vi "set current selections.vi"   [LabVIEW 2017, in "vs-tree-utility.lvlib" / "alias-tree.lvclass"]
uses:
  alias-tree.lvclass
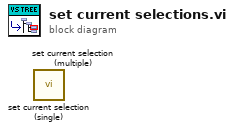
[diagram p0: block diagram]
diagram:
  n1 = call "set current selection (single).vi"() -> ()  [unwired: 9 in, 3 out]
  n2 = call "set current selection (multiple).vi"() -> ()  [unwired: 8 in, 4 out]
